vi "Initialize Device Core.vi"(8 "error in (no error)":errorcluster, 9 "Reset (F)":bool, 10 "Resource Name":string, 11 "CS++DeviceActor in":refnum<class "CS++DeviceActor.lvclass">) -> (0 "error out":errorcluster, 3 "CS++DeviceActor out":refnum<class "CS++DeviceActor.lvclass">)   [LabVIEW 2014, in "CS++DeviceActor.lvlib" / "CS++DeviceActor.lvclass"]
doc: "Initialize device driver."
uses:
  CS++DeviceActor.lvclass
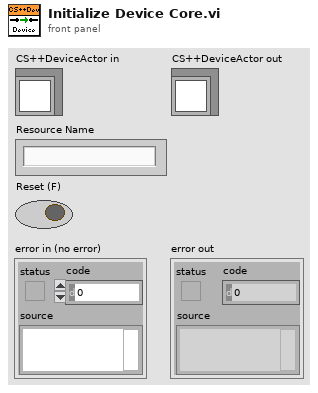
[diagram p1: front panel]
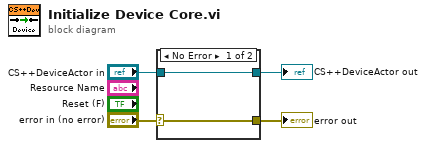
[diagram p0: block diagram]
diagram:
  n1 = case shown="No Error" "error in (no error)" {
    selector: "error in (no error)" -> [w5 w8]
    tunnel: [w5 w8] -> w3
    tunnel: [w6 w7] -> w1
    tunnel: "CS++DeviceActor in" -> [w6 w7]
    frame No Error {
    }
    frame Error {
    }
  }
  "error out" <- w3
  "CS++DeviceActor out" <- w1
